vi "Create Report Header.vi"(8 "error in (no error)":errorcluster, 9 "UUT.lvclass":refnum<class "UUT.lvclass">, 10 "Report in":refnum<class "Report.lvclass">, 11 "Sequence Engine in":refnum<class "Sequence Engine.lvclass">) -> (0 "error out":errorcluster, 2 "Report out":refnum<class "Report.lvclass">, 3 "Sequence Engine out":refnum<class "Sequence Engine.lvclass">)   [LabVIEW 2021, in "Sequence Engine.lvlib" / "Sequence Engine.lvclass"]
uses:
  Sequence Engine.lvclass
  PPLs/Report.lvlibp/Classes/Report/Report.lvclass
  UUT/UUT.lvclass
  PPLs/Report.lvlibp/Classes/Report/Report Metadata.ctl
  Sequence Engine.lvclass/Sequence Engine.ctl
  UUT/UUT.lvclass/UUT.ctl
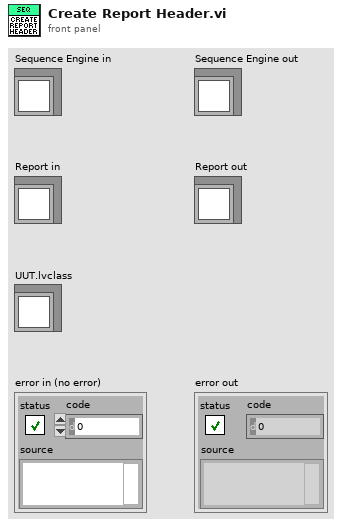
[diagram p1: front panel]
types:
  T1 = typedef "Report.lvlibp/Report.lvclass/Report Metadata.ctl" = cluster{"Model":string, "Serial Number":string, "Recipe Name":string, "Recipe Version":u16, "Username":string, "Test Status":string, "First Fail Test":string, "Start Time":timestamp, "Stop Time":timestamp, "Cycle Time (sec)":u16, "Execution Type":string}
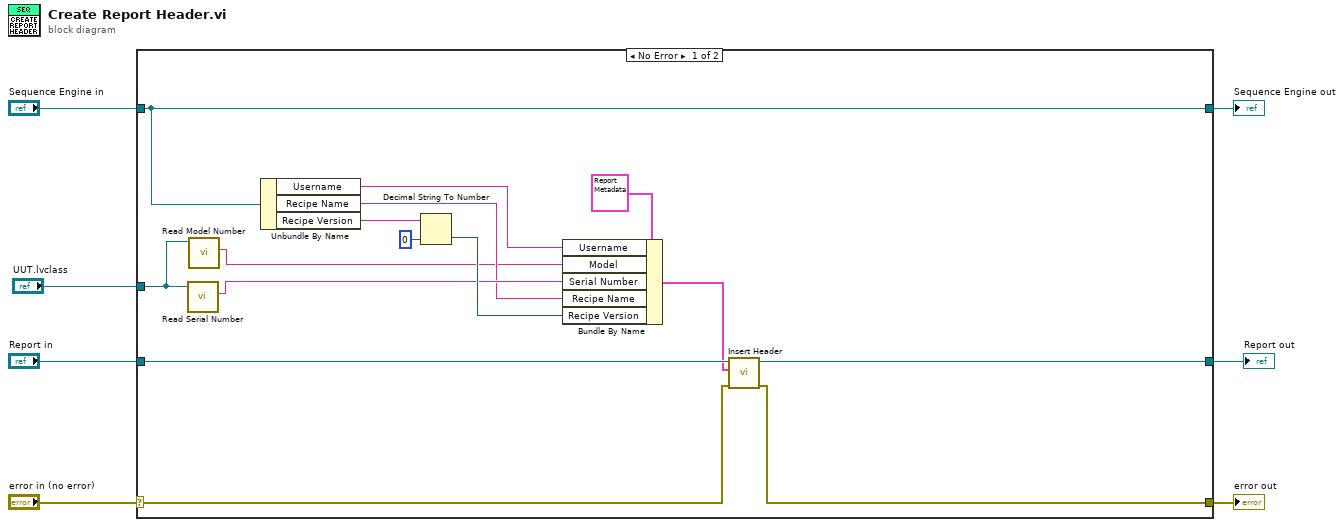
[diagram p0: block diagram]
diagram:
  n1 = case shown="No Error" "error in (no error)" {
    selector: "error in (no error)" -> [w18 w25]
    tunnel: [w17 w25] -> w6
    tunnel: [w22 w24] -> w4
    tunnel: "Sequence Engine in" -> [w22 w24]
    tunnel: "Report in" -> [w16 w23]
    tunnel: "UUT.lvclass" -> [w12 _]
    tunnel: [w14 w23] -> w1
    frame No Error {
      n2 = call "Read Serial Number.vi"("UUT in"=w12) -> ("Serial Number"=w15:string)  [unwired: 8 in, 2 out]
      n3 = call "Read Model Number.vi"("UUT in"=w12) -> ("Model Number"=w11:string)  [unwired: 8 in, 2 out]
      n4 = Unbundle By Name(w22) -> ("Username"=w8:string, "Recipe Name"=w13:string, "Recipe Version"=w21:string)
      n5 = Decimal String To Number(string=w21, default (0L)=u16 0 ("default (0 I32)")) -> (number=w20:u16)  [unwired: 1 in, 1 out]
      n6 = Bundle By Name(cluster=T1 {"Model"="", "Serial Number"="", "Recipe Name"="", "Recipe Version"=0, "Username"="", "Test Status"="", "First Fail Test"="", "Start Time"=timestamp(0 s since 1904-01-01), "Stop Time"=timestamp(0 s since 1904-01-01), "Cycle Time (sec)"=0, "Execution Type"=""} ("Report Metadata"), "Username"=w8, "Model"=w11, "Serial Number"=w15, "Recipe Name"=w13, "Recipe Version"=w20) -> (w9:T1)
      n7 = call "Insert Header.vi"("error in (no error)"=w18, "Report Metadata"=w9, "Report in"=w16) -> ("error out"=w17:errorcluster, "Report out"=w14:refnum<class "Report.lvclass">)  [unwired: 7 in]
    }
    frame Error {
    }
  }
  "error out" <- w6
  "Sequence Engine out" <- w4
  "Report out" <- w1
